vi "Format VI Info Column.vi"(8 "error in (no error)":errorcluster {"code" format="Error %.0f"}, 9 "Column":T9=enum."FP", 10 "VI Info":T1, 11 "VIDoc Printer - Confluence In":refnum<class "VIDoc Printer - Confluence.lvclass">) -> (0 "error out":errorcluster {"code" format="Error %.0f"}, 1 "Header":string, 2 "Cell Text":string, 3 "VIDoc Printer - Confluence Out":refnum<class "VIDoc Printer - Confluence.lvclass">, 4 "Viable Value?":bool, 5 "Pixel Width":i16=275)   [LabVIEW 2023, in "VIDoc Printer - Confluence.lvlib" / "VIDoc Printer - Confluence.lvclass"]
uses:
  VIDoc Printer - Confluence.lvclass
  C:/projects/DMC/Tooling/Git-Action-Service/Source/Documentation Generation/Printers/Printer/VIDoc Printer.lvclass
  Settings/Confluence Printer Settings/VI Info Column.ctl
  Parsing/TypeDefs/Method Spec Cluster.ctl
  Parsing/TypeDefs/VI Type Extended Enum.ctl
  <vilib>/picture/picture.llb/imagedata.ctl
  Parsing/TypeDefs/Class Dispatch Type Enum.ctl
  Parsing/TypeDefs/Controls Info Cluster.ctl
  <vilib>/Utility/miscctls.llb/LVKeyTypeDef.ctl
  <vilib>/Utility/miscctls.llb/LVPointTypeDef.ctl
  Parsing/SubVIs/Structure Reporter/Tree Cluster.ctl
  Types/VI Info Image Types.ctl
  Printer/VIDoc Printer.lvclass/VIDoc Printer.ctl
  Printer/Accessors/Get Formatting Settings - Bookmark Options.vi
  Printer/Accessors/Get Formatting Settings.vi
  Accessors/Get Current Page Title.vi
  <userlib>/_PetranWay/LabVIEW Confluence API/Source/Confluence/HTML/Add Link to Text/Add URL to Text.vi
  VIDoc Printer - Confluence.lvclass/VIDoc Printer - Confluence.ctl
  Printer/VIDoc Printer.lvclass
  Confluence Formatting/Confluence Formatting.lvlib
  <userlib>/_PetranWay/LabVIEW Confluence API/Source/PetranWay_Confluence API.lvlib
  Settings/Confluence Printer Settings/VIDoc Settings - Confluence.lvclass
  Parsing/VIDoc Parsing.lvlib
  Parsing/SubVIs/Structure Reporter/Structure Reporter.lvlib
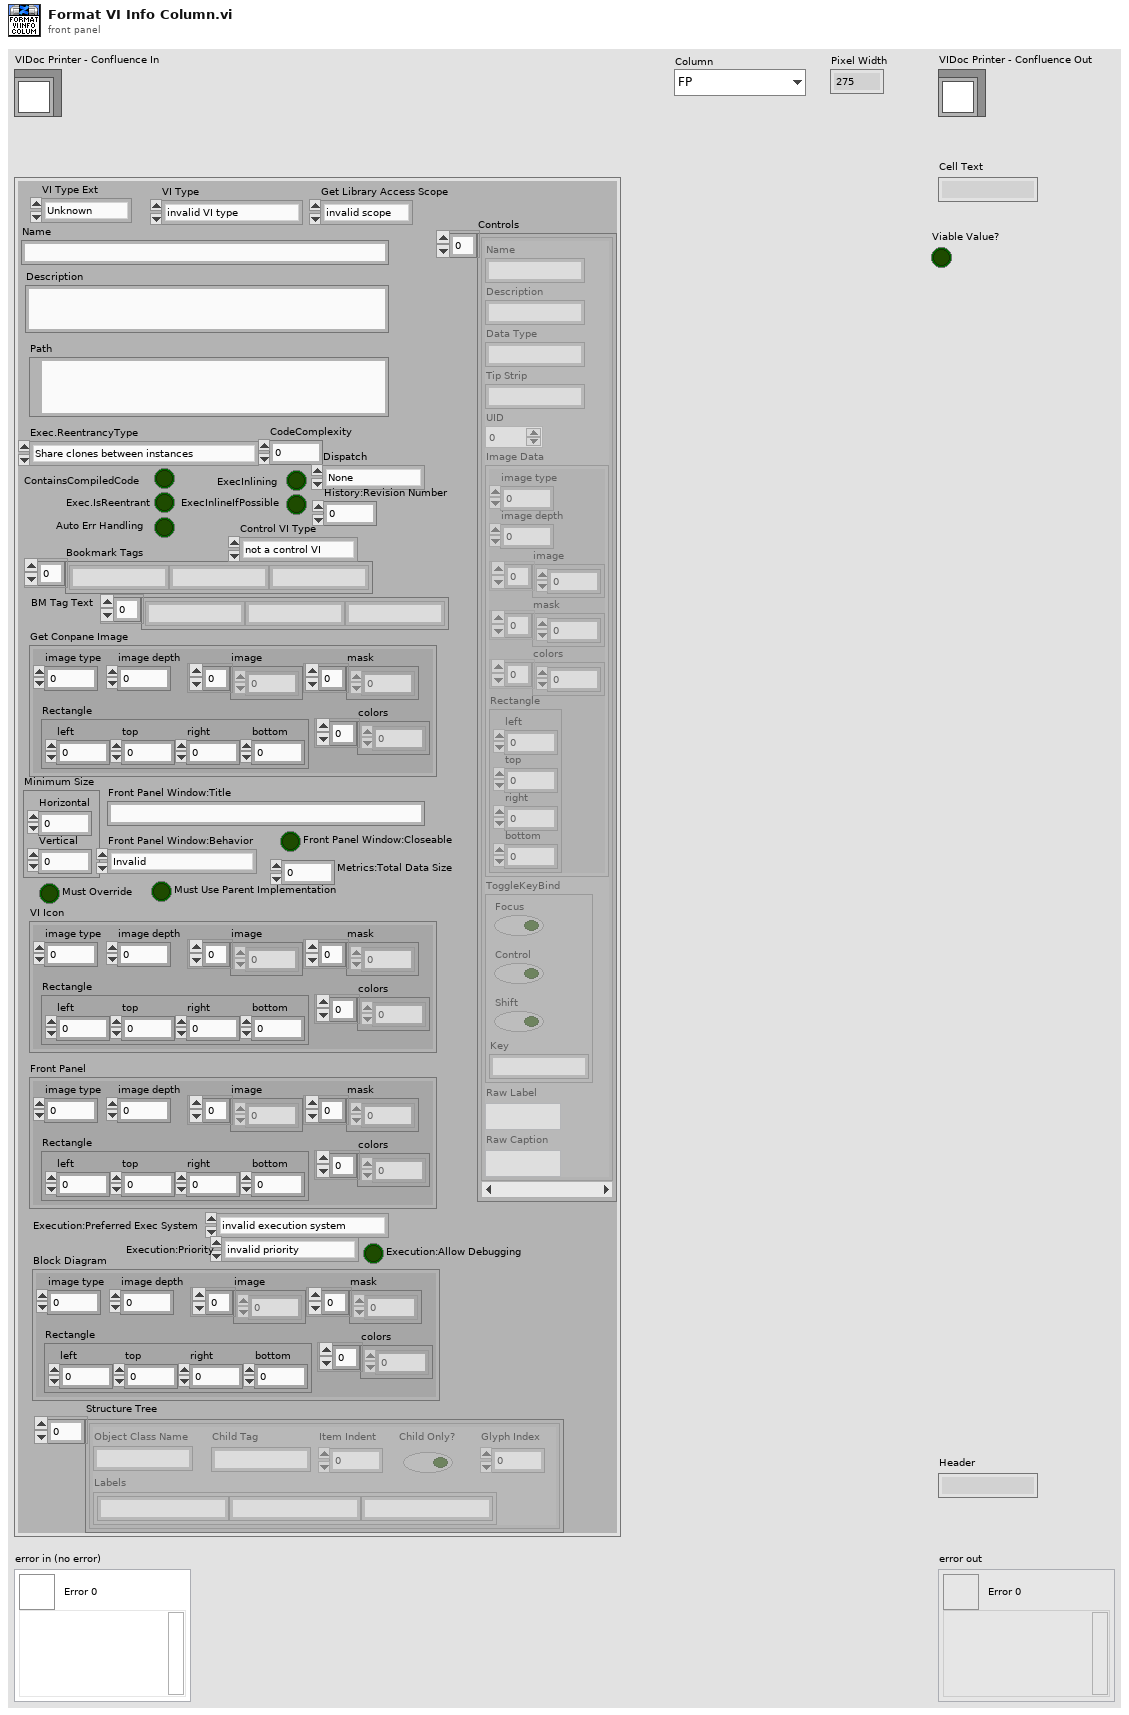
[diagram p1: front panel]
types:
  T1 = typedef "VIDoc Parsing.lvlib/Method Spec Cluster.ctl" = cluster{"VI Type Ext":T2, "Name":string, "Path":path, "Get Conpane Image":T3, "Description":string, "Get Library Access Scope":enum32{"invalid scope", "public", "private", "protected", "community"}, "Dispatch":T4, "ContainsCompiledCode":bool, "Exec.IsReentrant":bool, "Exec.ReentrancyType":enum16{"Share clones between instances", "Preallocate clone for each instance"}, "ExecInlining":bool, "ExecInlineIfPossible":bool, "Auto Err Handling":bool, "CodeComplexity":sgl, "Bookmark Tags":string[], "Control VI Type":enum32{"not a control VI", "control", "typedef", "strict typedef"}, "Controls":T5[], "VI Type":enum32{"invalid VI type", "Standard VI", "Control VI", "Global VI", "Polymorphic VI", "Configuration VI", "SubSystem", "Facade VI", "Method VI", "Statechart Diagram VI"}, "Minimum Size":T7, "Front Panel Window:Title":string, "Front Panel Window:Behavior":enum32{"Invalid", "Default", "Floating", "Floating/Auto-Hide", "Modal"}, "Front Panel Window:Closeable":bool, "Must Override":bool, "Must Use Parent Implementation":bool, "VI Icon":T3, "Front Panel":T3, "History:Revision Number":u32, "Metrics:Total Data Size":u32, "Execution:Allow Debugging":bool, "Execution:Preferred Exec System":enum32{"invalid execution system", "user interface", "standard", "instrument i/o", "data acquisition", "other 1", "other 2", "same as caller"}, "Execution:Priority":enum32{"invalid priority", "background priority", "normal priority", "above normal priority", "high priority", "time critical priority", "subroutine"}, "BM Tag Text":string[], "Block Diagram":T3, "Structure Tree":T8[]}
  T2 = typedef "VIDoc Parsing.lvlib/VI Type Extended Enum.ctl" = enum16{"Unknown", "Class Method", "Class Accessor Get", "Class Accessor Set", "Class Control", "Library Method", "Library Control", "VI", "Control"}
  T3 = typedef "imagedata.ctl" = cluster{"image type":i32, "image depth":i32, "image":u8[], "mask":u8[], "colors":u32[], "Rectangle":cluster{"left":i16, "top":i16, "right":i16, "bottom":i16}}
  T4 = typedef "VIDoc Parsing.lvlib/Class Dispatch Type Enum.ctl" = enum16{"None", "Static", "Dynamic"}
  T5 = typedef "VIDoc Parsing.lvlib/Controls Info Cluster.ctl" = cluster{"Name":string, "Description":string, "Data Type":string, "Tip Strip":string, "UID":i32, "Image Data":T3, "ToggleKeyBind":T6, "Raw Label":string, "Raw Caption":string}
  T6 = typedef "LVKeyTypeDef.ctl" = cluster{"Focus":bool, "Control":bool, "Shift":bool, "Key":string}
  T7 = typedef "LVPointTypeDef.ctl" = cluster{"Horizontal":i16, "Vertical":i16}
  T8 = typedef "VIDoc Parsing.lvlib/Structure Reporter.lvlib/Tree Cluster.ctl" = cluster{"Object Class Name":string, "Labels":string[], "Child Tag":string, "Item Indent":i32, "Child Only?":bool, "Glyph Index":i32}
  T9 = typedef "VIDoc Printer - Confluence.lvlib/VIDoc Settings - Confluence.lvclass/VI Info Column.ctl" = enum16{"Name", "Conpane", "BD", "FP", "VI Icon", "Description", "Reentrant", "Inline", "Auto Error", "Compiled", "Code Complexity", "Data Size", "Debug", "Priority", "Rev", "Minimum Size", "Title", "FP Behavior", "FP Closeable", "Author", "Commit Hash", "Last Change", "Branch", "Scope", "Type", "Dispatch", "Must Override", "Must Use Parent", "Structure Tree"}
  T10 = typedef "VIDoc Printer - Confluence.lvlib/VIDoc Printer - Confluence.lvclass/VI Info Image Types.ctl" = enum16{"Conpane", "FP", "BD", "Icon"}
  T11 = typedef "VIDoc Printer.lvlib/Printer Settings.lvclass/Bookmark Options.ctl" = cluster{"Bookmarks as New Line in VI Descriptions":bool, "Unique Bookmark Tags Only":bool, "Include Tag and Text":bool}
  T12 = enum16{"Share clones between instances", "Preallocate clone for each instance"}
  T13 = typedef "VIDoc Printer.lvlib/Printer Settings.lvclass/Formatting Options.ctl" = cluster{"Background":cluster{"Public Scope":T14, "Protected Scope":T14, "Community Scope":T14, "Private Scope":T14, "Unknown Scope":T14, "Auto Error Handling":T14, "Inline":T14, "Separate CC":T14, "Execution Priority Normal":T14, "Reentrancy Non-RE":T14}, "Bookmark Options":T11}
  T14 = typedef "VIDoc Printer.lvlib/Printer Settings.lvclass/Background Formatting Cluster.ctl" = cluster{"Option":bool, "Color":u32, "Operator":bool}
  T15 = enum32{"invalid priority", "background priority", "normal priority", "above normal priority", "high priority", "time critical priority", "subroutine"}
  T16 = enum32{"Invalid", "Default", "Floating", "Floating/Auto-Hide", "Modal"}
  T17 = cluster{"Timestamp":timestamp, "Commit Hash":string, "Author Name":string, "Branch":string, "Commit Hash URL":string}
  T18 = enum32{"invalid scope", "public", "private", "protected", "community"}
  T19 = enum32{"not a control VI", "control", "typedef", "strict typedef"}
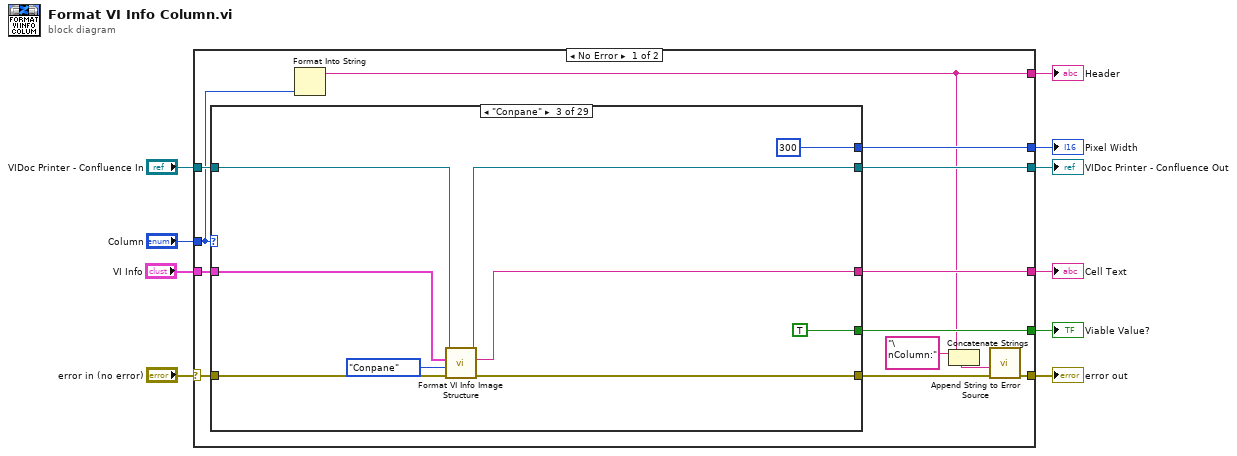
[diagram p0: block diagram]
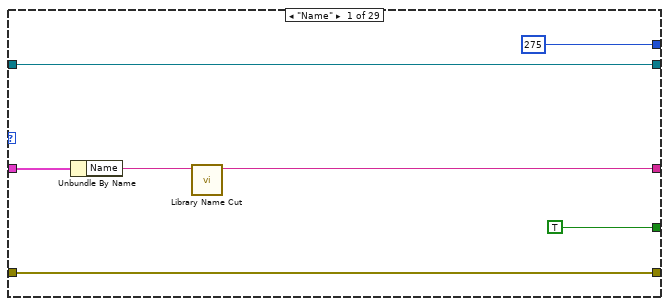
[diagram p2: hidden frame]
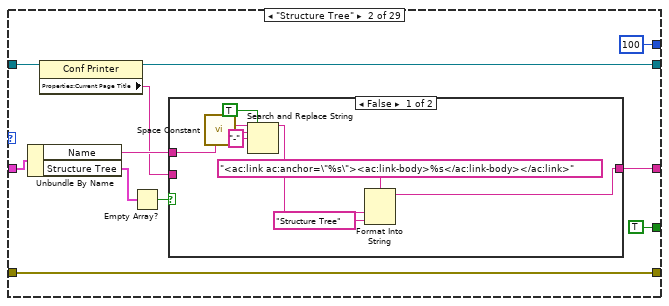
[diagram p3: hidden frame]
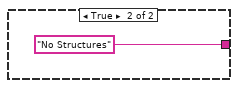
[diagram p4: hidden frame]
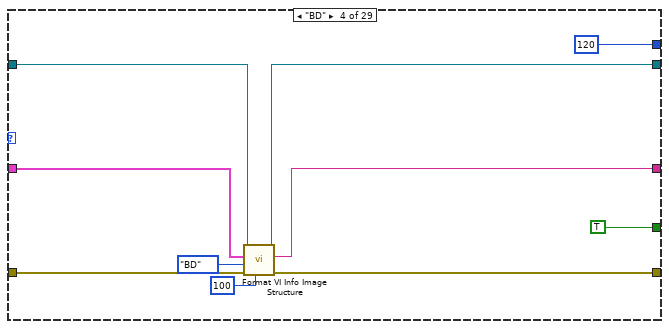
[diagram p5: hidden frame]
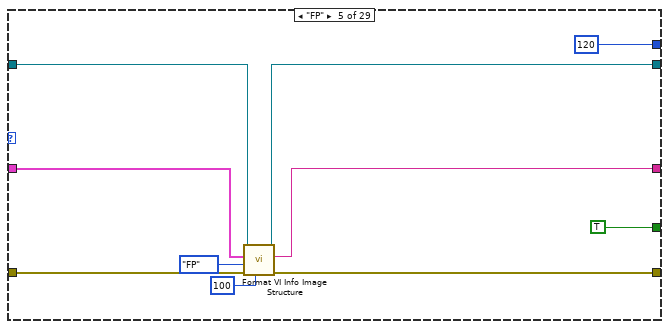
[diagram p6: hidden frame]
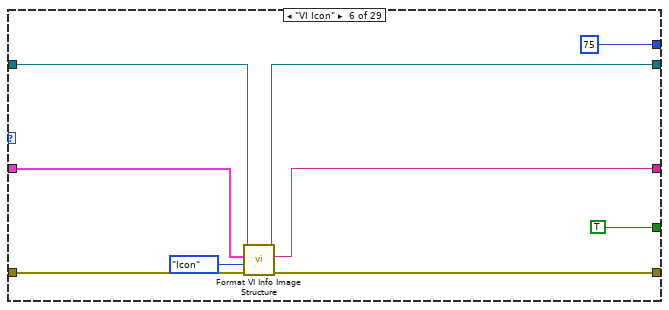
[diagram p7: hidden frame]
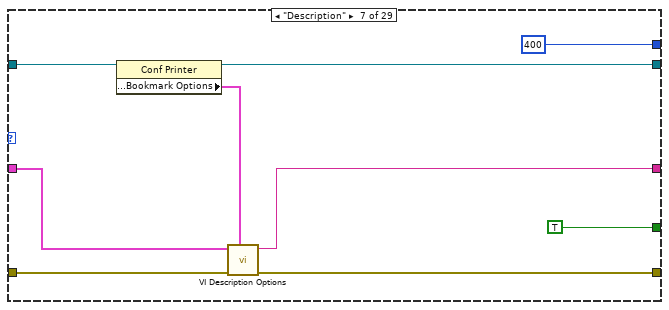
[diagram p8: hidden frame]
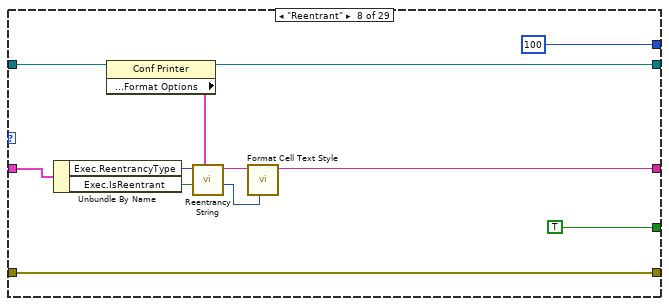
[diagram p9: hidden frame]
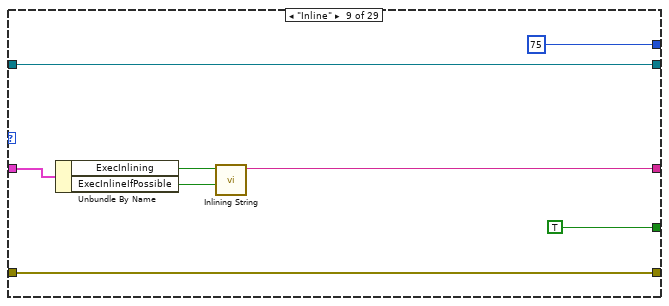
[diagram p10: hidden frame]
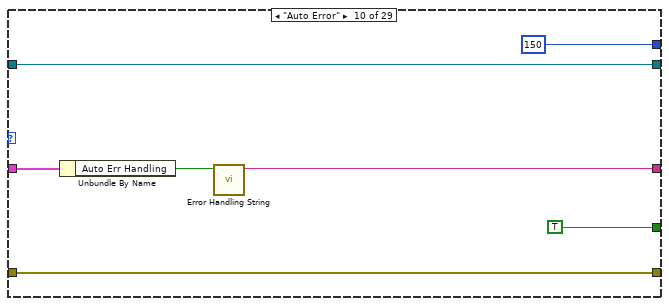
[diagram p11: hidden frame]
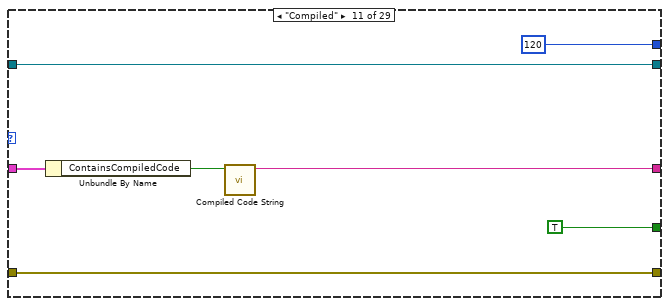
[diagram p12: hidden frame]
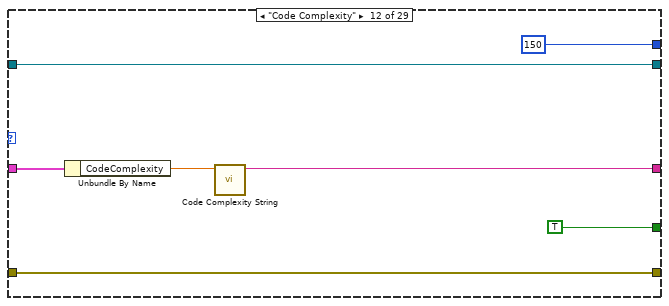
[diagram p13: hidden frame]
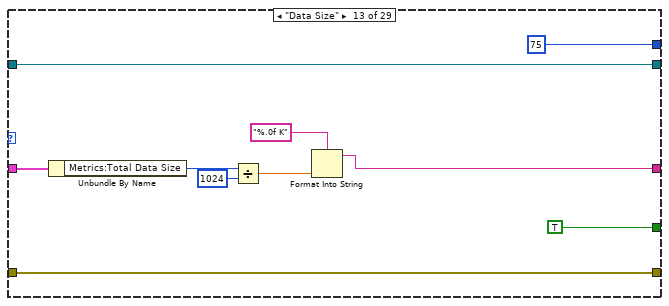
[diagram p14: hidden frame]
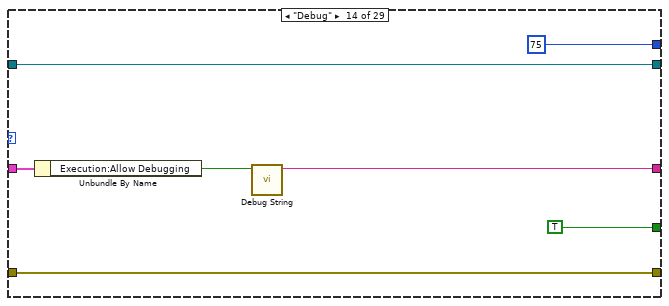
[diagram p15: hidden frame]
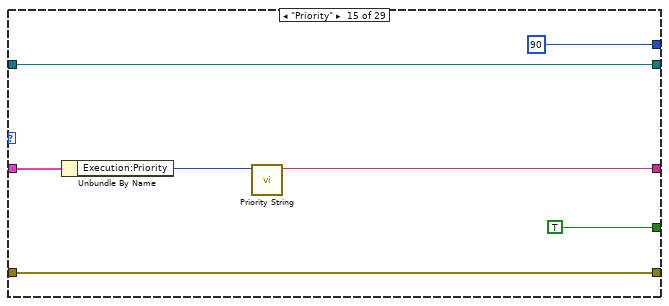
[diagram p16: hidden frame]
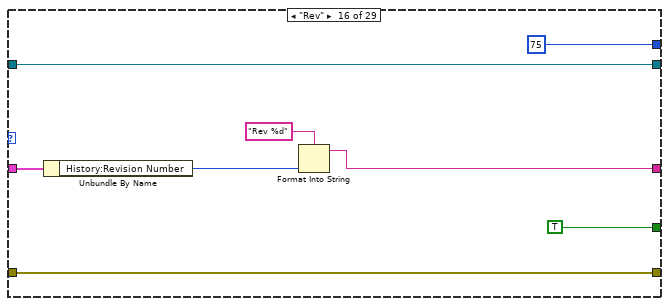
[diagram p17: hidden frame]
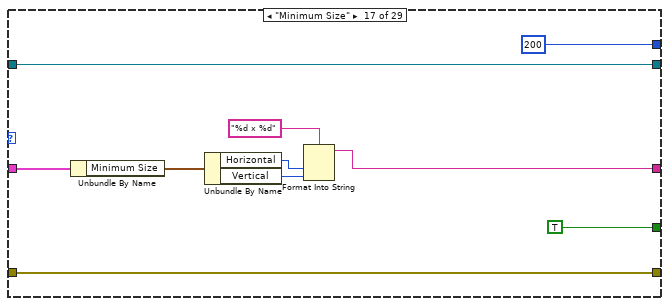
[diagram p18: hidden frame]
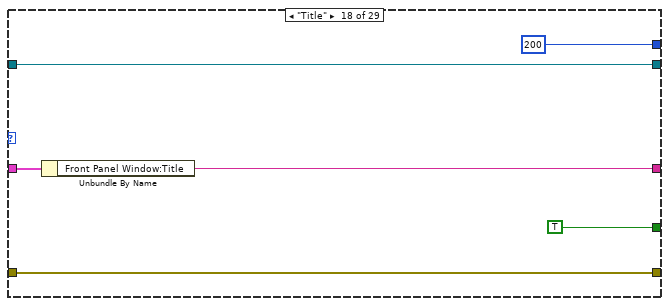
[diagram p19: hidden frame]
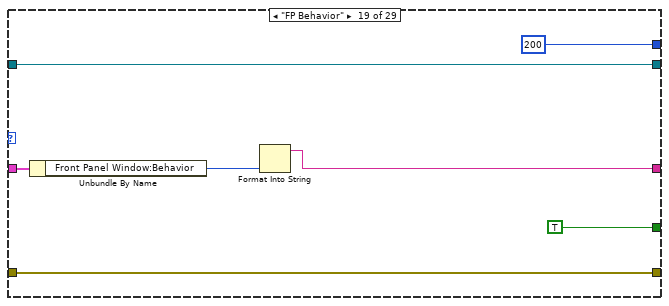
[diagram p20: hidden frame]
diagram:
  n1 = case shown="No Error" "error in (no error)" {
    selector: "error in (no error)" -> [w22 w292]
    tunnel: [w14 w292] -> w9
    tunnel: [w21 w291] -> w7
    tunnel: "VIDoc Printer - Confluence In" -> [w20 w291]
    tunnel: "Column" -> [w17 _]
    tunnel: "VI Info" -> [w19 _]
    tunnel: [w18 _] -> w4
    tunnel: [w12 _] -> w3
    tunnel: [w16 _] -> w2
    tunnel: [w15 FALSE ("File Change Info Available?")] -> w1
    frame No Error {
      n2 = case shown="\"Conpane\"" w17 {
        tunnel: [w30 w40 w55 w65 w75 w84 w90 w103 w114 w121 w128 w135 w145 w152 w159 w167 w177 w183 w190 w199 w210 w213 w242 w252 w261 w268 w272 w279 w286] -> w23
        tunnel: w22 -> [w30 w40 w58 w68 w78 w87 w95 w103 w114 w121 w128 w135 w145 w152 w159 w167 w177 w183 w190 w199 w209 w223 w241 w251 w261 w268 w272 w279 w286]
        tunnel: [w29 w32 w56 w66 w76 w85 w94 w107 w116 w123 w130 w137 w147 w154 w161 w169 w179 w185 w192 w201 w208 w222 w240 w250 w260 w267 w274 w281 w288] -> w21
        tunnel: w20 -> [w29 w41 w57 w67 w77 w86 w96 w108 w116 w123 w130 w137 w147 w154 w161 w169 w179 w185 w192 w201 w207 w221 w239 w249 w260 w267 w274 w281 w288]
        tunnel: w19 -> [w28 w39 w52 w62 w72 w81 w92 w106 w115 w122 w129 w136 w146 w153 w160 w168 w178 w184 w191 w200 w211 w224 w243 w253 w259 w266 w273 w280 w287]
        tunnel: [w25 w35 w54 w64 w74 w83 w91 w99 w111 w119 w126 w133 w140 w150 w157 w164 w172 w182 w188 w195 w204 w214 w234 w246 w255 w262 w269 w276 w283] -> w18
        tunnel: [i16 275 ("Pixel Width") i16 100 ("Pixel Width") i16 300 ("Pixel Width") i16 120 ("Pixel Width") i16 120 ("Pixel Width") i16 75 ("Pixel Width") i16 400 ("Pixel Width") i16 100 ("Pixel Width") i16 75 ("Pixel Width") i16 150 ("Pixel Width") i16 120 ("Pixel Width") i16 150 ("Pixel Width") i16 75 ("Pixel Width") i16 75 ("Pixel Width") i16 90 ("Pixel Width") i16 75 ("Pixel Width") i16 200 ("Pixel Width") i16 200 ("Pixel Width") i16 200 ("Pixel Width") i16 120 ("Pixel Width") i16 120 ("Pixel Width") i16 120 ("Pixel Width") i16 200 ("Pixel Width") i16 200 ("Pixel Width") i16 100 ("Pixel Width") i16 300 ("Pixel Width") i16 90 ("Pixel Width") i16 90 ("Pixel Width") i16 90 ("Pixel Width")] -> w16
        tunnel: [TRUE ("File Change Info Available?") TRUE ("File Change Info Available?") TRUE ("File Change Info Available?") TRUE ("File Change Info Available?") TRUE ("File Change Info Available?") TRUE ("File Change Info Available?") TRUE ("File Change Info Available?") TRUE ("File Change Info Available?") TRUE ("File Change Info Available?") TRUE ("File Change Info Available?") TRUE ("File Change Info Available?") TRUE ("File Change Info Available?") TRUE ("File Change Info Available?") TRUE ("File Change Info Available?") TRUE ("File Change Info Available?") TRUE ("File Change Info Available?") TRUE ("File Change Info Available?") TRUE ("File Change Info Available?") TRUE ("File Change Info Available?") TRUE ("File Change Info Available?") TRUE ("File Change Info Available?") w219 w233 w245 TRUE ("File Change Info Available?") TRUE ("File Change Info Available?") TRUE ("File Change Info Available?") TRUE ("File Change Info Available?") TRUE ("File Change Info Available?")] -> w15
        frame "Name" {
          n3 = Unbundle By Name(w28) -> ("Name"=w27:string)
          n4 = call "Library Name Cut.vi"("Name in"=w27) -> ("Name out"=w25:string)  [unwired: 10 in]
        }
        frame "Structure Tree" {
          n5 = Unbundle By Name(w39) -> ("Name"=w33:string, "Structure Tree"=w34:T8[])
          n6 = property class="Conf Printer"(reference=w41) -> (reference out=w32:refnum<class "VIDoc Printer - Confluence.lvclass">, "Properties:Current Page Title"=w31:string)  [unwired: 1 in, 1 out]
          n7 = Empty Array?(array=w34) -> (empty?=w36:bool)
          n8 = case shown="False" w36 {
            tunnel: [w43 "No Structures"] -> w35
            tunnel: w33 -> [w47 _]
            tunnel: w31 -> [_ _]
            frame False {
              n9 = call <vilib>:"Space Constant.vi"() -> ("String"=w49:string)
              n10 = Search and Replace String(replace all?=TRUE ("replace all? (F)"), input string=w47, search string=w49, replace string="-" ("replace string (\"\")")) -> (result string=w45:string)  [unwired: 4 in, 3 out]
              n11 = Format Into String(format string="<ac:link ac:anchor=\"%s\"><ac:link-body>%s</ac:link-body></ac:link>", w45, "Structure Tree" ("input 2")) -> (resulting string=w43:string)  [unwired: 2 in, 1 out]
            }
            frame True {
            }
          }
        }
        frame "Conpane" {
          n12 = call "Format VI Info Image Structure.vi"("Error in"=w58, "Image Type"=VI_Info_Image_Types."Conpane", "VI Info"=w52, "VIDoc Printer - Confluence In"=w57) -> ("Error out"=w55:errorcluster, "Image Structure Text"=w54:string, "VIDoc Printer - Confluence Out"=w56:refnum<class "VIDoc Printer - Confluence.lvclass">)  [unwired: 4 in, 1 out]
        }
        frame "BD" {
          n13 = call "Format VI Info Image Structure.vi"("Max Width (500 pixels)"=i16 100, "Error in"=w68, "Image Type"=VI_Info_Image_Types."BD", "VI Info"=w62, "VIDoc Printer - Confluence In"=w67) -> ("Error out"=w65:errorcluster, "Image Structure Text"=w64:string, "VIDoc Printer - Confluence Out"=w66:refnum<class "VIDoc Printer - Confluence.lvclass">)  [unwired: 3 in, 1 out]
        }
        frame "FP" {
          n14 = call "Format VI Info Image Structure.vi"("Max Width (500 pixels)"=i16 100, "Error in"=w78, "Image Type"=VI_Info_Image_Types."FP", "VI Info"=w72, "VIDoc Printer - Confluence In"=w77) -> ("Error out"=w75:errorcluster, "Image Structure Text"=w74:string, "VIDoc Printer - Confluence Out"=w76:refnum<class "VIDoc Printer - Confluence.lvclass">)  [unwired: 3 in, 1 out]
        }
        frame "VI Icon" {
          n15 = call "Format VI Info Image Structure.vi"("Error in"=w87, "Image Type"=VI_Info_Image_Types."Icon", "VI Info"=w81, "VIDoc Printer - Confluence In"=w86) -> ("Error out"=w84:errorcluster, "Image Structure Text"=w83:string, "VIDoc Printer - Confluence Out"=w85:refnum<class "VIDoc Printer - Confluence.lvclass">)  [unwired: 4 in, 1 out]
        }
        frame "Description" {
          n16 = property class="Conf Printer"(reference=w96) -> (reference out=w94:refnum<class "VIDoc Printer - Confluence.lvclass">, "Properties:Settings:Formatting Options:Bookmark Options"=w93:T11)  [unwired: 1 in, 1 out]
          n17 = call "VI Description Options.vi"("Bookmark Options"=w93, "Error in"=w95, "VI Info"=w92) -> ("Error out"=w90:errorcluster, "Description"=w91:string)  [unwired: 7 in]
        }
        frame "Reentrant" {
          n18 = Unbundle By Name(w106) -> ("Exec.ReentrancyType"=w105:T12, "Exec.IsReentrant"=w104:bool)
          n19 = property class="Conf Printer"(reference=w108) -> (reference out=w107:refnum<class "VIDoc Printer - Confluence.lvclass">, "Properties:Settings:Formatting Options:Format Options"=w100:T13)  [unwired: 1 in, 1 out]
          n20 = call "Reentrancy String.vi"("Format Options"=w100, "Exec.IsReentrant"=w104, "Exec.ReentrancyType"=w105) -> ("Cell Color"=w101:u32, "Reentrancy"=w102:string)  [unwired: 7 in]
          n21 = call "Format Cell Text Style.vi"("BG Color (Unchanged)"=w101, "String"=w102) -> ("Formatted Text"=w99:string)  [unwired: 8 in, 1 out]
        }
        frame "Inline" {
          n22 = Unbundle By Name(w115) -> ("ExecInlining"=w113:bool, "ExecInlineIfPossible"=w112:bool)
          n23 = call "Inlining String.vi"("ExecInlineIfPossible"=w112, "ExecInlining"=w113) -> ("Inline Text"=w111:string)  [unwired: 9 in]
        }
        frame "Auto Error" {
          n24 = Unbundle By Name(w122) -> ("Auto Err Handling"=w120:bool)
          n25 = call "Error Handling String.vi"("Auto Err Handling"=w120) -> ("Error Handling String"=w119:string)  [unwired: 10 in]
        }
        frame "Compiled" {
          n26 = Unbundle By Name(w129) -> ("ContainsCompiledCode"=w127:bool)
          n27 = call "Compiled Code String.vi"("ContainsCompiledCode"=w127) -> ("Compiled Code String"=w126:string)  [unwired: 10 in]
        }
        frame "Code Complexity" {
          n28 = Unbundle By Name(w136) -> ("CodeComplexity"=w134:sgl)
          n29 = call "Code Complexity String.vi"("CodeComplexity"=w134) -> ("Code Complexity String"=w133:string)  [unwired: 10 in]
        }
        frame "Data Size" {
          n30 = Unbundle By Name(w146) -> ("Metrics:Total Data Size"=w141:u32)
          n31 = Divide(x=w141, y=u32 1024) -> (x/y=w142:dbl)
          n32 = Format Into String(format string="%.0f K", w142) -> (resulting string=w140:string)  [unwired: 2 in, 1 out]
        }
        frame "Debug" {
          n33 = Unbundle By Name(w153) -> ("Execution:Allow Debugging"=w151:bool)
          n34 = call "Debug String.vi"("Allow Debugging"=w151) -> ("Debug String"=w150:string)  [unwired: 10 in]
        }
        frame "Priority" {
          n35 = Unbundle By Name(w160) -> ("Execution:Priority"=w158:T15)
          n36 = call "Priority String.vi"("Execution:Priority"=w158) -> ("Priority String"=w157:string)  [unwired: 10 in]
        }
        frame "Rev" {
          n37 = Unbundle By Name(w168) -> ("History:Revision Number"=w165:u32)
          n38 = Format Into String(format string="Rev %d", w165) -> (resulting string=w164:string)  [unwired: 2 in, 1 out]
        }
        frame "Minimum Size" {
          n39 = Unbundle By Name(w178) -> ("Minimum Size"=w173:T7)
          n40 = Unbundle By Name(w173) -> ("Horizontal"=w176:i16, "Vertical"=w175:i16)
          n41 = Format Into String(format string="%d x %d", w176, w175) -> (resulting string=w172:string)  [unwired: 2 in, 1 out]
        }
        frame "Title" {
          n42 = Unbundle By Name(w184) -> ("Front Panel Window:Title"=w182:string)
        }
        frame "FP Behavior" {
          n43 = Unbundle By Name(w191) -> ("Front Panel Window:Behavior"=w189:T16)
          n44 = Format Into String(w189) -> (resulting string=w188:string)  [unwired: 3 in, 1 out]
        }
        frame "FP Closeable" {
          n45 = Unbundle By Name(w200) -> ("Front Panel Window:Closeable"=w198:bool)
          n46 = Select(t="Closable" ("format string"), s=w198, f="Not Closable" ("format string")) -> (s? t:f=w195:string)
        }
        frame "Author" {
          n47 = Unbundle By Name(w211) -> ("Path"=w206:path)
          n48 = call "Retrieve File Change Info.vi"("error in (no error)"=w209, "Absolute File Path"=w206, "VIDoc Printer - Confluence In"=w207) -> ("error out"=w210:errorcluster, "File Change Info"=w205:T17, "VIDoc Printer - Confluence Out"=w208:refnum<class "VIDoc Printer - Confluence.lvclass">)  [unwired: 5 in, 1 out]
          n49 = Unbundle By Name(w205) -> ("Author Name"=w204:string)
        }
        frame "Commit Hash" {
          n50 = Unbundle By Name(w224) -> ("Path"=w220:path)
          n51 = call "Retrieve File Change Info.vi"("error in (no error)"=w223, "Absolute File Path"=w220, "VIDoc Printer - Confluence In"=w221) -> ("error out"=w216:errorcluster, "File Change Info Available?"=w219:bool, "File Change Info"=w215:T17, "VIDoc Printer - Confluence Out"=w222:refnum<class "VIDoc Printer - Confluence.lvclass">)  [unwired: 5 in]
          n52 = Unbundle By Name(w215) -> ("Commit Hash"=w218:string, "Commit Hash URL"=w217:string)
          n53 = case shown="\"\"" w217 {
            selector: w217 -> [_ w230]
            tunnel: w218 -> [w227 w232]
            tunnel: [w227 w231] -> w214
            tunnel: w216 -> [w226 w229]
            tunnel: [w226 w228] -> w213
            frame "" {
            }
            frame Default {
              n54 = call-poly <userlib>:"Add Link to Text.vi"("Text"=w232, "URL"=w230, "error in (no error)"=w229) -> ("HTML Text String"=w231:string, "error out"=w228:errorcluster)  [unwired: 10 in, 1 out]
            }
          }
        }
        frame "Last Change" {
          n55 = Unbundle By Name(w243) -> ("Path"=w238:path)
          n56 = call "Retrieve File Change Info.vi"("error in (no error)"=w241, "Absolute File Path"=w238, "VIDoc Printer - Confluence In"=w239) -> ("error out"=w242:errorcluster, "File Change Info Available?"=w233:bool, "File Change Info"=w237:T17, "VIDoc Printer - Confluence Out"=w240:refnum<class "VIDoc Printer - Confluence.lvclass">)  [unwired: 5 in]
          n57 = Unbundle By Name(w237) -> ("Timestamp"=w236:timestamp)
          n58 = Format Into String(format string="%<%Y/%m/%d %H:%M:%S>T", w236) -> (resulting string=w234:string)  [unwired: 2 in, 1 out]
        }
        frame "Branch" {
          n59 = Unbundle By Name(w253) -> ("Path"=w248:path)
          n60 = call "Retrieve File Change Info.vi"("error in (no error)"=w251, "Absolute File Path"=w248, "VIDoc Printer - Confluence In"=w249) -> ("error out"=w252:errorcluster, "File Change Info Available?"=w245:bool, "File Change Info"=w247:T17, "VIDoc Printer - Confluence Out"=w250:refnum<class "VIDoc Printer - Confluence.lvclass">)  [unwired: 5 in]
          n61 = Unbundle By Name(w247) -> ("Branch"=w246:string)
        }
        frame "Scope" {
          n62 = Unbundle By Name(w259) -> ("Get Library Access Scope"=w256:T18)
          n63 = call "Scope String.vi"("Get Library Access Scope"=w256) -> ("String"=w255:string)  [unwired: 10 in]
        }
        frame "Type" {
          n64 = Unbundle By Name(w266) -> ("Control VI Type"=w263:T19)
          n65 = call "Control Type to String.vi"("Control VI Type"=w263) -> ("String"=w262:string)  [unwired: 10 in]
        }
        frame "Dispatch" {
          n66 = Unbundle By Name(w273) -> ("Dispatch"=w270:T4)
          n67 = Format Into String(w270) -> (resulting string=w269:string)  [unwired: 3 in, 1 out]
        }
        frame "Must Override" {
          n68 = Unbundle By Name(w280) -> ("Must Override"=w277:bool)
          n69 = Format Into String(w277) -> (resulting string=w276:string)  [unwired: 3 in, 1 out]
        }
        frame "Must Use Parent" {
          n70 = Unbundle By Name(w287) -> ("Must Use Parent Implementation"=w284:bool)
          n71 = Format Into String(w284) -> (resulting string=w283:string)  [unwired: 3 in, 1 out]
        }
      }
      n72 = Format Into String(w17) -> (resulting string=w12:string)  [unwired: 3 in, 1 out]
      n73 = Concatenate Strings("\nColumn:" ("string"), w12) -> (w11:string)
      n74 = call "Append String to Error Source.vi"("Error In"=w23, "String to Append"=w11) -> ("Error Out"=w14:errorcluster)  [unwired: 9 in]
    }
    frame Error {
    }
  }
  "error out" <- w9
  "VIDoc Printer - Confluence Out" <- w7
  "Pixel Width" <- w2
  "Cell Text" <- w4
  "Header" <- w3
  "Viable Value?" <- w1
